vi "Get TableDefinitionPart.vi"(7 "Sheet Name":string, 8 "error in":errorcluster, 10 "Table Name":string, 11 "SpreadsheetDoc in":refnum<k24>) -> (0 "error out":errorcluster, 2 "TableDefinitionPart":refnum<k24>, 3 "SpreadsheetDo out":refnum<k24>, 5 "Sheet Name":string)   [LabVIEW 2019, in "Open Xml.lvlib"]
uses:
  Open Xml.lvlib
  D:/git/Open-Xml-LabVIEW/Source/DocumentFormat.OpenXml.dll
  DocumentFormat.OpenXml.dll
  D:/git/Open-Xml-LabVIEW/Source/OpenXmlGenericsWrapper.dll
  OpenXmlGenericsWrapper.dll
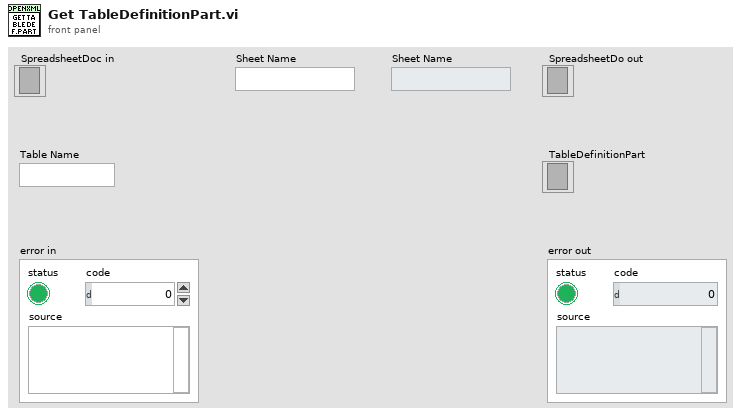
[diagram p1: front panel]
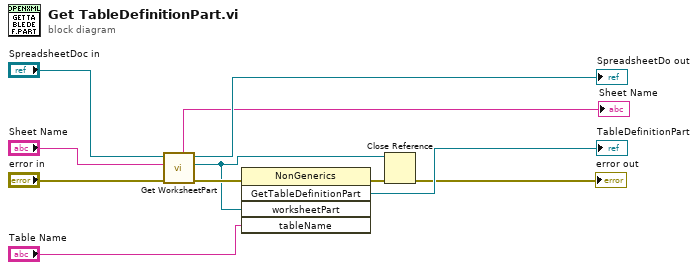
[diagram p0: block diagram]
diagram:
  n1 = call "Get WorksheetPart.vi"("error in"="error in", "Sheet Name"="Sheet Name", "SpreadsheetDocument in"="SpreadsheetDoc in") -> ("error out"=w8:errorcluster, "WorksheetPart"=w2:refnum<k24>, "SpreadsheetDocument out"=→"SpreadsheetDo out":refnum<k24>, "SheetName"=→"Sheet Name":string)  [unwired: 5 in]
  n2 = invoke class="NonGenerics" method="GetTableDefinitionPart"(error in=w8, "worksheetPart"=w2, "tableName"="Table Name") -> (error out=w5:errorcluster, "GetTableDefinitionPart"=→"TableDefinitionPart":refnum<k24>)  [unwired: 2 in, 3 out]
  n3 = Close Reference(reference=w2, error in (no error)=w5) -> (error out=→"error out":errorcluster)
